vi "Timing Waveform Generator.vi"() -> ()   [LabVIEW 2017]
uses:
  <vilib>/DAQmx/configure/timing.llb/DAQmx Timing (Implicit).vi
  <vilib>/DAQmx/configure/trigger.llb/DAQmx Start Trigger (Digital Edge).vi
  <resource>/objmgr/daqmx.rc
  <vilib>/Utility/error.llb/DialogType.ctl
  <vilib>/DAQmx/create/channels.llb/DAQmx Create Channel (CO-Pulse Generation-Time).vi
  <vilib>/DAQmx/create/channels.llb/DAQmx Create Channel (CO-Pulse Generation-Ticks).vi
  Controls/Translation Stage Types.ctl
  Hardware/Table Stage/Controls/Translation Stage Cluster.ctl
  Controls/System Parameters.ctl
panel:
  in  "Stop 2":bool
  in  "Pulse Duration":dbl=1.0 format="%.6f"
  in  "Output Terminal":tag="/Dev1/PFI12"
  in  "Trigger Type":enum32{"No Trigger", "Digital Start"}(tab)
  in  "Retriggerable":bool
  in  "Edge":i32(ring)=10280 items=["Rising"=10280, "Falling"=10171]
  in  "Digital Trigger Source":tag
  in  "Counter":tag="Dev1/ctr0"
  in  "Stop":bool
  in  "System Parameters [In]":T1={"Vibratome"={"Z Bottom [mm]"=0.0, "Pre Cut Dwell [s]"=0.0, "Blade Frequency [RPM]"=0, "Slice Speed [mm/s]"=0.0, "Post Cut Dwell [s]"=0.0, "Ramp Time [s]"=0.0, "Start X [mm]"=0.0, "Start Y [mm]"=0.0, "Slice Length [mm]"=0.0, "Slice Axis"=enum."Y Axis", "Controller VISA Ref"="COM4"}, "Table Stages"={"X Stage"={"Position"=0.0, "Is.Enabled?"=FALSE, "Is.Connected?"=FALSE, "Device SN"="45876539", "AccelerationMaximum"=0.0, "VelocityMaximum"=0.0, "Acceleration"=0.0, "Velocity"=0.0, "waitTimeout (ms)"=0, "Model"=enum."None", "Is.Homed?"=FALSE}, "Y Stage"={"Position"=0.0, "Is.Enabled?"=FALSE, "Is.Connected?"=FALSE, "Device SN"="45876539", "AccelerationMaximum"=0.0, "VelocityMaximum"=0.0, "Acceleration"=0.0, "Velocity"=0.0, "waitTimeout (ms)"=0, "Model"=enum."None", "Is.Homed?"=FALSE}, "Z Stage"={"Position"=0.0, "Is.Enabled?"=FALSE, "Is.Connected?"=FALSE, "Device SN"="45876539", "AccelerationMaximum"=0.0, "VelocityMaximum"=0.0, "Acceleration"=0.0, "Velocity"=0.0, "waitTimeout (ms)"=0, "Model"=enum."None", "Is.Homed?"=FALSE}}}
  # "To configure and use a trigger you must have the necessary tab selected above."
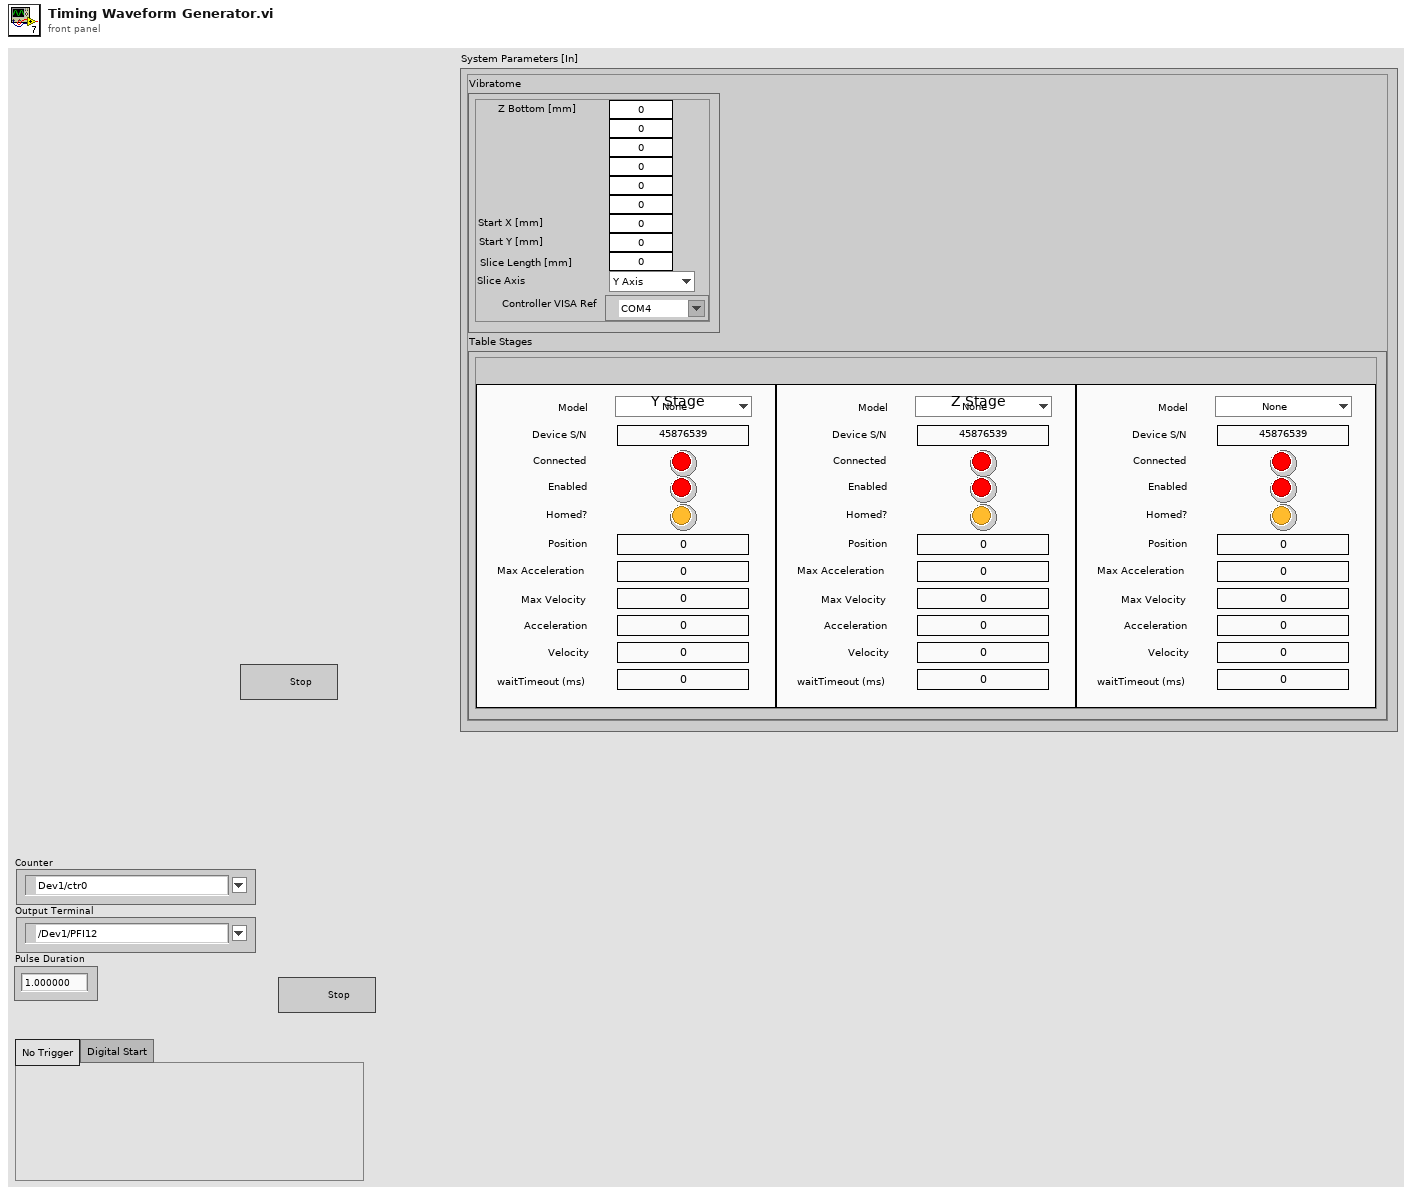
[diagram p1: front panel]
types:
  T1 = typedef "System Parameters.ctl" = cluster{"Vibratome":cluster{"Z Bottom [mm]":dbl, "Pre Cut Dwell [s]":dbl, "Blade Frequency [RPM]":u16, "Slice Speed [mm/s]":dbl, "Post Cut Dwell [s]":dbl, "Ramp Time [s]":dbl, "Start X [mm]":dbl, "Start Y [mm]":dbl, "Slice Length [mm]":dbl, "Slice Axis":enum16{"X Axis", "Y Axis", "Z Axis"}, "Controller VISA Ref":refnum<visa-resource-name>}, "Table Stages":cluster{"X Stage":T2, "Y Stage":T2, "Z Stage":T2}}
  T2 = typedef "Translation Stage Cluster.ctl" = cluster{"Position":dbl, "Is.Enabled?":bool, "Is.Connected?":bool, "Device SN":string, "AccelerationMaximum":dbl, "VelocityMaximum":dbl, "Acceleration":dbl, "Velocity":dbl, "waitTimeout (ms)":i32, "Model":T3, "Is.Homed?":bool}
  T3 = typedef "Translation Stage Types.ctl" = enum16{"None", "Thorlabs LTS", "Thorlabs MLJ"}
  T4 = typedef "DialogType.ctl" = u16
  T5 = enum16{"32 x 32", "64 x 64", "128 x 128", "256 x 256", "512 x 512", "1024 x 1024", "2048 x 2048"}
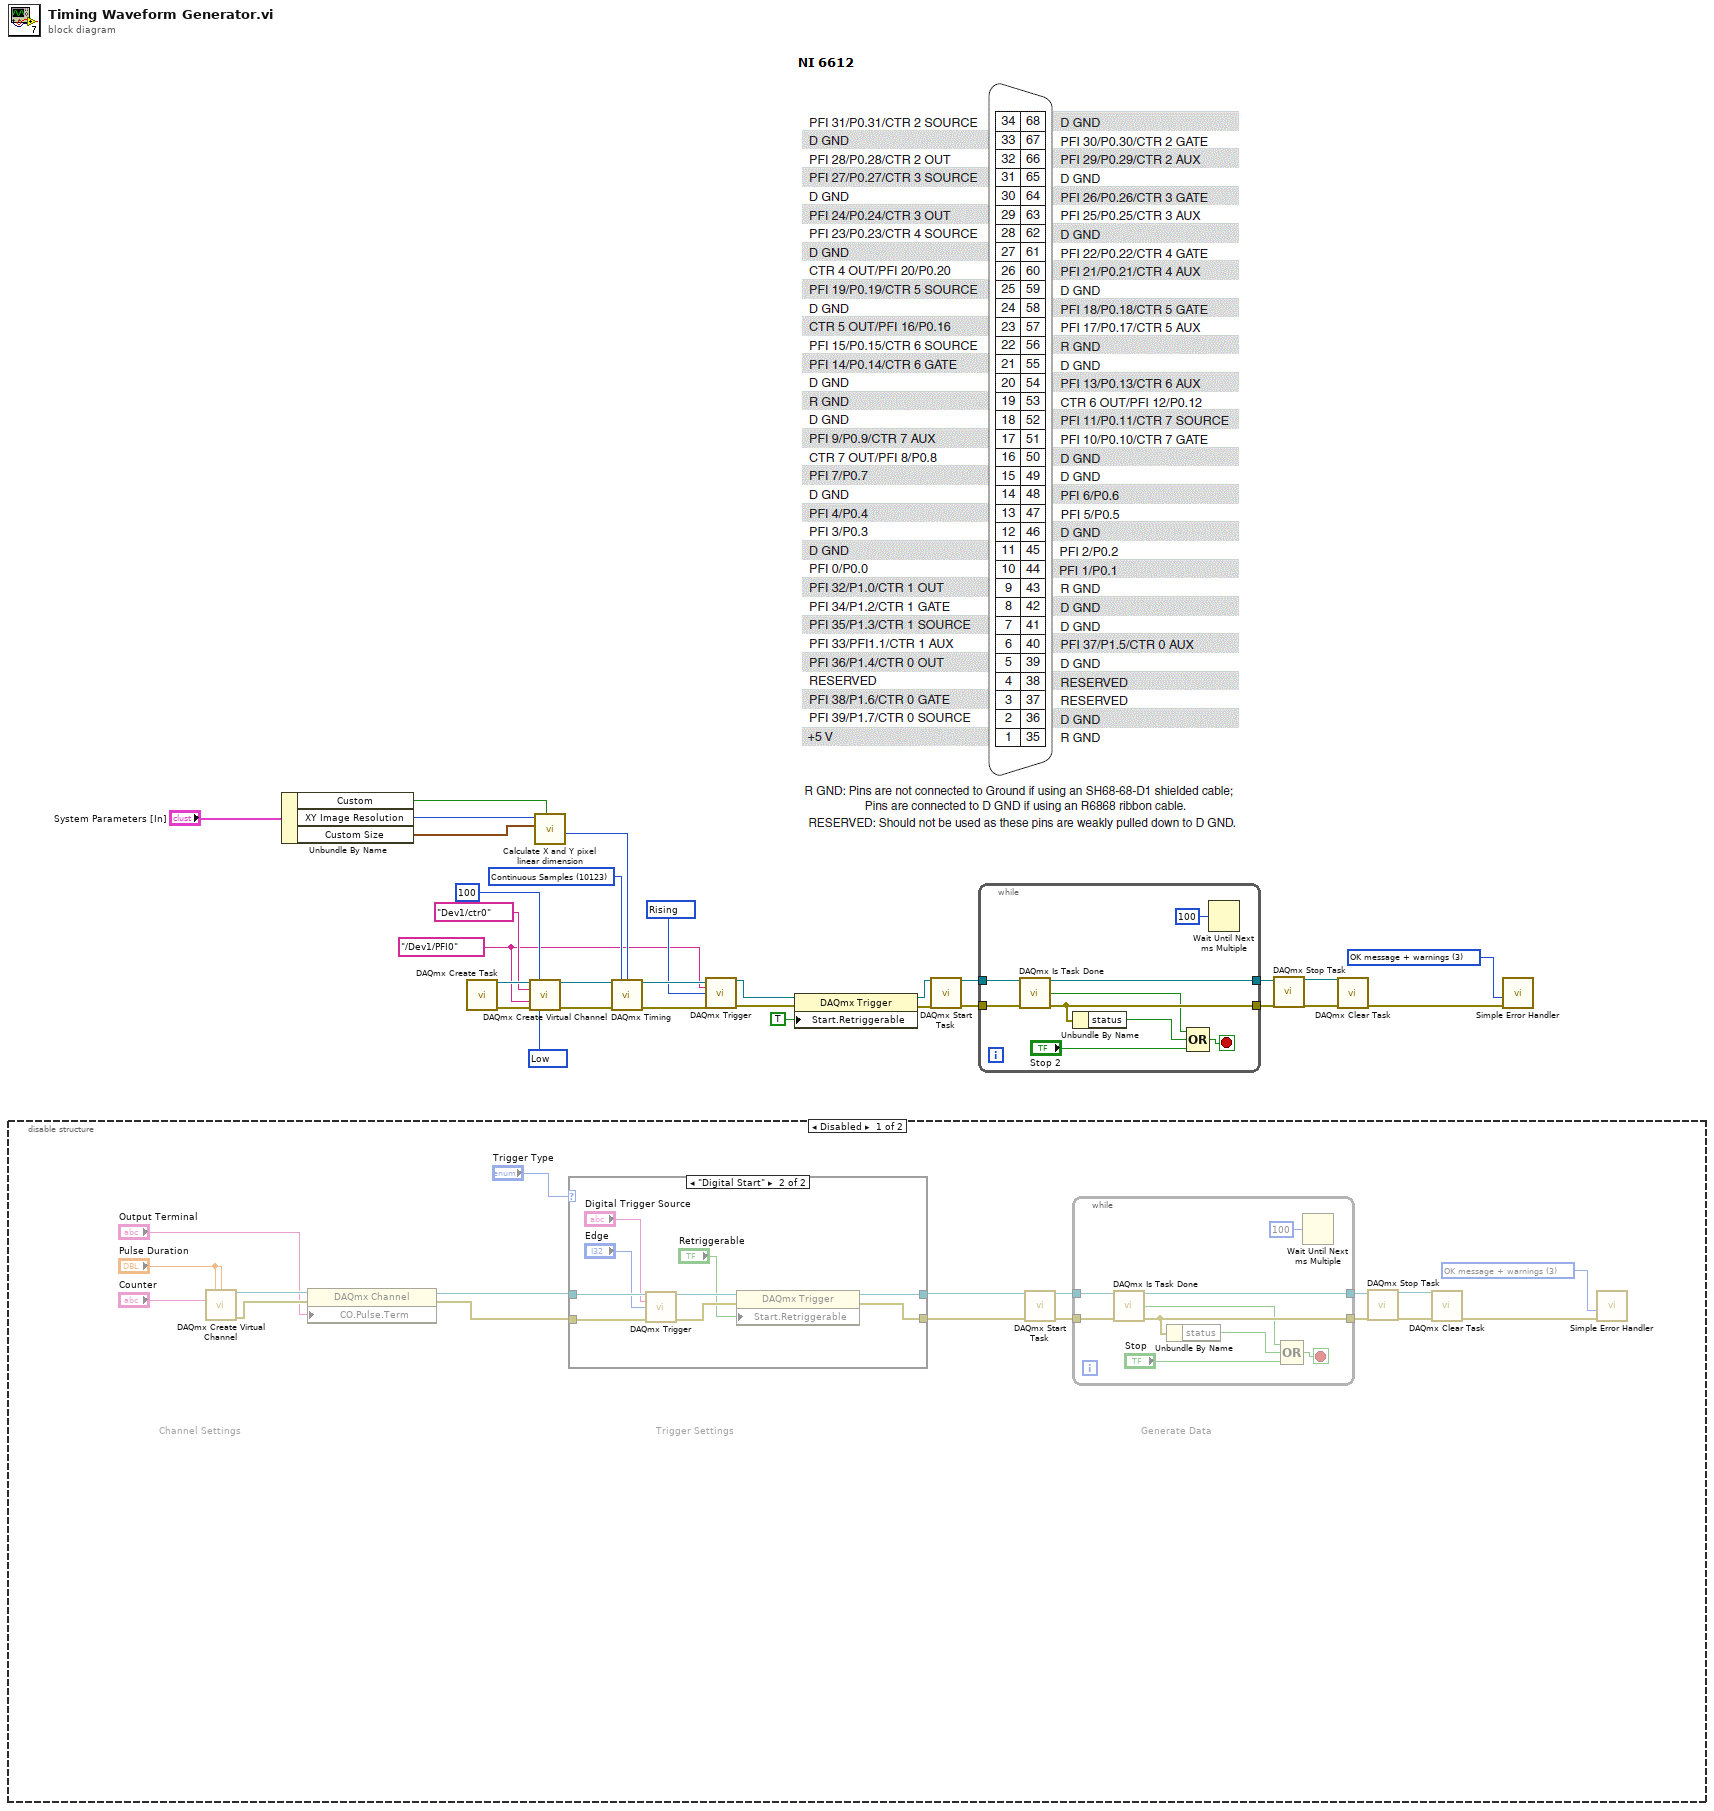
[diagram p0: block diagram]
diagram:
  w10 = T4 3 items=["no dialog", "OK message", "continue or stop message", "OK message + warnings", "continue/stop + warnings"] ("type of dialog (OK msg:1)")
  w14 = tag "/Dev1/PFI0" ("source of ticks")
  w15 = 10214 items=["High"=10192, "Low"=10214] ("idle state")
  w18 = 10280 items=["Rising"=10280, "Falling"=10171] ("edge")
  w26 = 10123 items=["Finite Samples"=10178, "Continuous Samples"=10123, "Hardware Timed Single Point"=12522] ("sample mode")
  n1 = disable-structure shown="Disabled" {
    frame Disabled {
      w31 = T4 3 items=["no dialog", "OK message", "continue or stop message", "OK message + warnings", "continue/stop + warnings"] ("type of dialog (OK msg:1)")
      # "Generate Data"
      # "Trigger Settings"
      # "Channel Settings"
      n2 = call-poly <vilib>:"DAQmx Create Virtual Channel.vi"("high time"="Pulse Duration", "low time"="Pulse Duration", "counter"="Counter") -> ("task out"=w41:refnum<k21>, "error out"=w40:errorcluster)  [unwired: 11 in]
      n3 = property class="DAQmx Channel"(reference=w41, error in=w40, "CO.Pulse.Term"="Output Terminal") -> (reference out=w37:refnum<k21>, error out=w38:errorcluster)
      n4 = case shown="\"Digital Start\"" "Trigger Type" {
        tunnel: w37 -> [w59 w68]
        tunnel: w38 -> [w58 w67]
        tunnel: [w59 w64] -> w42
        tunnel: [w58 w63] -> w43
        frame "No Trigger", Default {
        }
        frame "Digital Start" {
          n5 = call-poly <vilib>:"DAQmx Trigger.vi"("task/channels in"=w68, "source"="Digital Trigger Source", "edge"="Edge", "error in"=w67) -> ("task out"=w61:refnum<k21>, "error out"=w62:errorcluster)  [unwired: 10 in]
          n6 = property class="DAQmx Trigger"(reference=w61, error in=w62, "Start.Retriggerable"="Retriggerable") -> (reference out=w64:refnum<k21>, error out=w63:errorcluster)
        }
      }
      n7 = call <vilib>:"DAQmx Start Task.vi"("task/channels in"=w42, "error in"=w43) -> ("task out"=w48:refnum<k21>, "error out"=w47:errorcluster)  [unwired: 12 in]
      n8 = while {
        tunnel: w48 -> [w57]
        tunnel: w47 -> [w56]
        tunnel: [w53] -> w34
        tunnel: [w54] -> w35
        stop <- w55 stop-if-true
        n9 = call <vilib>:"DAQmx Is Task Done.vi"("task/channels in"=w57, "error in"=w56) -> ("task out"=w54:refnum<k21>, "task done?"=w49:bool, "error out"=w53:errorcluster)  [unwired: 11 in]
        n10 = Unbundle By Name(w53) -> ("status"=w52:bool)
        n11 = Compound Arithmetic op=OR(w49, w52, "Stop") -> (w55:bool)
        n12 = Wait Until Next ms Multiple(millisecond multiple=u32 100) -> ()  [unwired: 1 out]
      }
      n13 = call <vilib>:"DAQmx Stop Task.vi"("task/channels in"=w35, "error in"=w34) -> ("task out"=w33:refnum<k21>, "error out"=w32:errorcluster)  [unwired: 12 in]
      n14 = call <vilib>:"DAQmx Clear Task.vi"("task in"=w33, "error in"=w32) -> ("error out"=w46:errorcluster)  [unwired: 13 in]
      n15 = call <vilib>:"Simple Error Handler.vi"("type of dialog (OK msg:1)"=w31, "error in (no error)"=w46) -> ()  [unwired: 3 in, 5 out]
    }
    frame Enabled {
    }
  }
  n16 = Unbundle By Name("System Parameters [In]") -> ("Custom"=w29:bool, "XY Image Resolution"=w28:T5, "Custom Size"=w27:cluster{"X":u16, "Y":u16})
  n17 = call <vilib>:"DAQmx Create Task.vi"() -> ("task out"=w22:refnum<k21>, "error out"=w24:errorcluster)  [unwired: 14 in]
  n18 = call-poly <vilib>:"DAQmx Create Virtual Channel.vi"("task in"=w22, "high ticks"=u32 100, "counter"=tag "Dev1/ctr0", "source of ticks"=w14, "error in"=w24, "idle state"=w15) -> ("task out"=w21:refnum<k21>, "error out"=w23:errorcluster)  [unwired: 8 in]
  n19 = call "Calculate X and Y pixel linear dimension.vi"("Imaging Parameter.Custom"=w29, "Custom Size"=w27, "XY Image Resolution"=w28) -> ("X Px Dim (FFOV)"=w25:u16)  [unwired: 5 in, 3 out]
  n20 = call-poly <vilib>:"DAQmx Timing.vi"("task/channels in"=w21, "sample mode"=w26, "samples per channel"=w25, "error in"=w23) -> ("task out"=w19:refnum<k21>, "error out"=w20:errorcluster)  [unwired: 10 in]
  n21 = call-poly <vilib>:"DAQmx Trigger.vi"("task/channels in"=w19, "source"=w14, "edge"=w18, "error in"=w20) -> ("task out"=w12:refnum<k21>, "error out"=w13:errorcluster)  [unwired: 10 in]
  n22 = property class="DAQmx Trigger"(reference=w12, error in=w13, "Start.Retriggerable"=TRUE) -> (reference out=w1:refnum<k21>, error out=w2:errorcluster)
  n23 = call <vilib>:"DAQmx Start Task.vi"("task/channels in"=w1, "error in"=w2) -> ("task out"=w3:refnum<k21>, "error out"=w4:errorcluster)  [unwired: 12 in]
  n24 = while {
    tunnel: w3 -> [w77]
    tunnel: w4 -> [w76]
    tunnel: [w73] -> w7
    tunnel: [w74] -> w6
    stop <- w75 stop-if-true
    n25 = call <vilib>:"DAQmx Is Task Done.vi"("task/channels in"=w77, "error in"=w76) -> ("task out"=w74:refnum<k21>, "task done?"=w69:bool, "error out"=w73:errorcluster)  [unwired: 11 in]
    n26 = Unbundle By Name(w73) -> ("status"=w72:bool)
    n27 = Compound Arithmetic op=OR(w69, w72, "Stop 2") -> (w75:bool)
    n28 = Wait Until Next ms Multiple(millisecond multiple=u32 100) -> ()  [unwired: 1 out]
  }
  n29 = call <vilib>:"DAQmx Stop Task.vi"("task/channels in"=w6, "error in"=w7) -> ("task out"=w8:refnum<k21>, "error out"=w9:errorcluster)  [unwired: 12 in]
  n30 = call <vilib>:"DAQmx Clear Task.vi"("task in"=w8, "error in"=w9) -> ("error out"=w5:errorcluster)  [unwired: 13 in]
  n31 = call <vilib>:"Simple Error Handler.vi"("type of dialog (OK msg:1)"=w10, "error in (no error)"=w5) -> ()  [unwired: 3 in, 5 out]
